vi "isRemoteControlServiceRunning.vi"(8 "error in (no error)":errorcluster, 11 "VGS_RemoteControlClient in":refnum<class "VGS_RemoteControlClient.lvclass">) -> (0 "error out":errorcluster, 2 "isRemoteControlServiceRunning":bool, 3 "VGS_RemoteControlClient out":refnum<class "VGS_RemoteControlClient.lvclass">)   [LabVIEW 2022 SP3, in "LV_VGS.lvlib" / "VGS_RemoteControlClient.lvclass"]
doc: "<B>Checks if a Remote Control Service is running and accessible. </B>\n\nThis method checks if the VG Remote Control Service is running on a specified computer and if the service is accessible. (i.e. if the firewall doesn't block the service).\n\nReturns\nThe method will return true if the service is accessible, otherwise, it will return false."
uses:
  VGS_RemoteControlClient.lvclass
  VGS_RemoteControlClient.lvclass/VGS_RemoteControlClient.ctl
  C:/Users/Andrey/Documents/GitHub/LV_VGS/vgs_project.dll
  vgs_project.dll
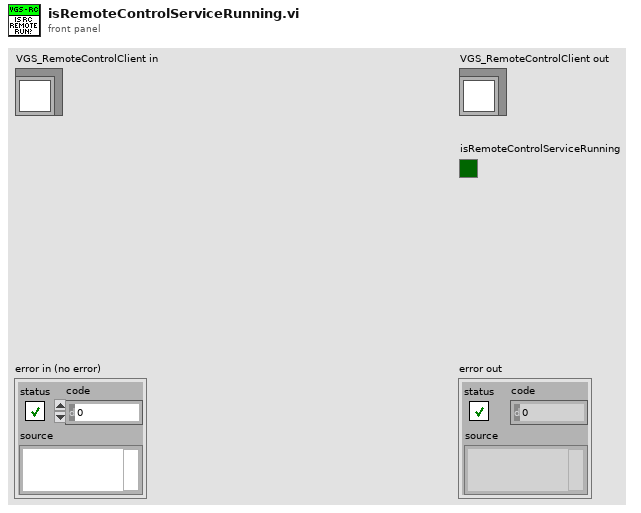
[diagram p1: front panel]
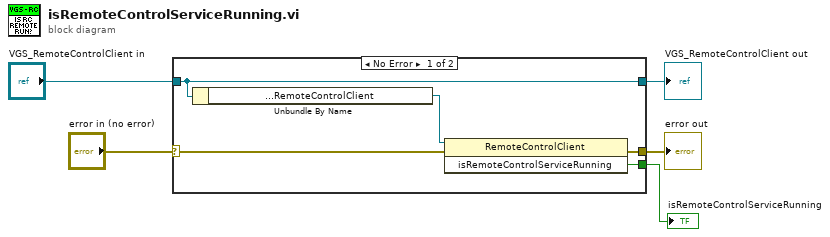
[diagram p0: block diagram]
diagram:
  n1 = case shown="No Error" "error in (no error)" {
    selector: "error in (no error)" -> [w8 w11]
    tunnel: [w7 w11] -> w4
    tunnel: [w10 w12] -> w2
    tunnel: "VGS_RemoteControlClient in" -> [w10 w12]
    tunnel: [w6 _] -> w1
    frame No Error {
      n2 = Unbundle By Name(w10) -> ("VGS.Project.Interop.RemoteControlClient"=w9:refnum<k24>)
      n3 = invoke class="RemoteControlClient" method="isRemoteControlServiceRunning"(reference=w9, error in=w8) -> (error out=w7:errorcluster, "isRemoteControlServiceRunning"=w6:bool)  [unwired: 1 in, 1 out]
    }
    frame Error {
    }
  }
  "error out" <- w4
  "VGS_RemoteControlClient out" <- w2
  "isRemoteControlServiceRunning" <- w1
